vi "orientacion.vi"(0 "COM Bluegiga in":refnum<visa-resource-name>, 5 "error in (no error)":errorcluster) -> (11 "Orientacion":u8, 14 "COM Bluegiga out":refnum<visa-resource-name>, 15 "Portrait":bool, 16 "Landscape":bool, 17 "Reverse Portrait":bool, 18 "Reverse Landscape":bool, 19 "error out":errorcluster)   [LabVIEW 2020]
panel:
  out "characteristic value":u8[](array[numeric])
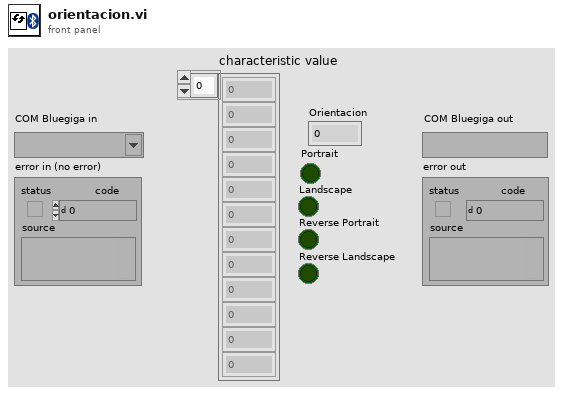
[diagram p1: front panel]
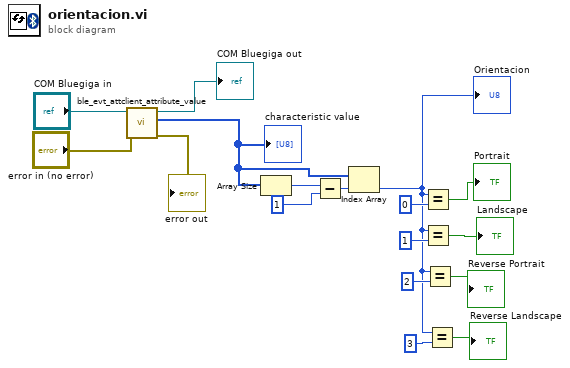
[diagram p0: block diagram]
diagram:
  n1 = call <vilib>:"ble_evt_attclient_attribute_value.vi"("error in (no error)"="error in (no error)", "COM Bluegiga in"="COM Bluegiga in") -> ("error out"=→"error out":errorcluster, "characteristic value"=w15:u8[], "COM Bluegiga out"=→"COM Bluegiga out":refnum<visa-resource-name>)  [unwired: 6 in, 1 out]
  "characteristic value" <- w15
  n2 = Array Size(array=w15) -> (size(s)=w10:i32)
  n3 = Subtract(x=w10, y=1) -> (x-y=w17:i32)
  n4 = Index Array(array=w15, index=w17) -> (element=w1:u8)
  "Orientacion" <- w1
  n5 = Equal?(x=w1, y=u8 0) -> (x = y?=→"Portrait":bool)
  n6 = Equal?(x=w1, y=u8 1) -> (x = y?=→"Landscape":bool)
  n7 = Equal?(x=w1, y=u8 2) -> (x = y?=→"Reverse Portrait":bool)
  n8 = Equal?(x=w1, y=u8 3) -> (x = y?=→"Reverse Landscape":bool)
